vi "User Bridge Control.vi"   [LabVIEW 2011]
uses:
  <vilib>/Rock Robotics/WPI/Solenoid/WPI_SolenoidValue.ctl
  <vilib>/Rock Robotics/WPI/Solenoid/WPI_SolenoidGetEnum.vi
  <vilib>/Rock Robotics/WPI/Solenoid/WPI_SolenoidSetEnum.vi
types:
  T1 = typedef "WPI_JoystickDevRef.ctl" = cluster{"Device":T2}
  T2 = typedef "WPI_JoystickDeviceEnum.ctl" = enum16{"USB 1", "USB 2", "USB 3", "USB 4", "Kinect 1", "Kinect 2"}
  T3 = typedef "WPI_SolenoidDevRef.ctl" = cluster{"DevStatus":errorcluster, "Solenoid Module":T4, "Forward Solenoid Channel":T5, "Reverse Solenoid Channel":T5}
  T4 = typedef "FPGA_TypedefSolenoidModule.ctl" = enum16{"Solenoid Module 1", "Solenoid Module 2"}
  T5 = typedef "WPI_SolenoidChannel.ctl" = enum8{"Solenoid 1", "Solenoid 2", "Solenoid 3", "Solenoid 4", "Solenoid 5", "Solenoid 6", "Solenoid 7", "Solenoid 8", "Invalid"}
  T6 = typedef "WPI_JoystickButtonState.ctl" = cluster{"Button 1":bool, "Button 2":bool, "Button 3":bool, "Button 4":bool, "Button 5":bool, "Button 6":bool, "Button 7":bool, "Button 8":bool, "Button 9":bool, "Button 10":bool, "Button 11":bool, "Button 12":bool}
  T7 = typedef "WPI_SolenoidValue.ctl" = enum16{"Off", "On", "Forward", "Reverse"}
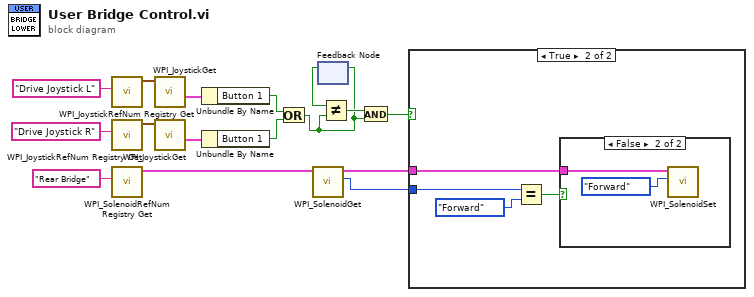
[diagram p0: block diagram]
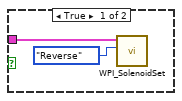
[diagram p3: hidden frame]
diagram:
  n1 = call <vilib>:"WPI_JoystickRefNum Registry Get.vi"("refnum name"="Drive Joystick L") -> ("JoystickDevRef"=w12:T1)  [unwired: 9 in, 1 out]
  n2 = call <vilib>:"WPI_JoystickRefNum Registry Get.vi"("refnum name"="Drive Joystick R") -> ("JoystickDevRef"=w15:T1)  [unwired: 9 in, 1 out]
  n3 = call <vilib>:"WPI_SolenoidRefNum Registry Get.vi"("refnum name"="Rear Bridge") -> ("SolenoidDevRef"=w3:T3)  [unwired: 9 in, 1 out]
  n4 = call <vilib>:"WPI_JoystickGet.vi"("JoystickDevRef"=w12) -> ("Buttons"=w10:T6)  [unwired: 4 in, 2 out]
  n5 = call <vilib>:"WPI_JoystickGet.vi"("JoystickDevRef"=w15) -> ("Buttons"=w14:T6)  [unwired: 4 in, 2 out]
  n6 = Unbundle By Name(w10) -> ("Button 1"=w9:bool)
  n7 = Unbundle By Name(w14) -> ("Button 1"=w8:bool)
  n8 = Or(x=w9, y=w8) -> (x .or. y?=w5:bool)
  n9 = call-poly <vilib>:"WPI_SolenoidGet.vi"("SolenoidDevRef"=w3) -> ("Value"=w1:T7, "SolenoidDevRef"=w2:T3)  [unwired: 8 in, 1 out]
  n10 = feedback-in #1(w5) -> ()
  n11 = feedback #1() -> (w7:bool)  [unwired: 1 in]
  n12 = Not Equal?(x=w7, y=w5) -> (x != y?=w6:bool)
  n13 = And(x=w6, y=w5) -> (x .and. y?=w4:bool)
  n14 = case shown="True" w4 {
    tunnel: w2 -> [_ w20]
    tunnel: w1 -> [_ w19]
    frame False {
    }
    frame True {
      n15 = Equal?(x=w19, y=WPI_SolenoidValue."Forward") -> (x = y?=w17:bool)
      n16 = case shown="False" w17 {
        tunnel: w20 -> [w22 w24]
        frame True {
          n17 = call-poly <vilib>:"WPI_SolenoidSet.vi"("Value"=WPI_SolenoidValue."Reverse", "SolenoidDevRef"=w22) -> ()  [unwired: 8 in, 2 out]
        }
        frame False {
          n18 = call-poly <vilib>:"WPI_SolenoidSet.vi"("Value"=WPI_SolenoidValue."Forward", "SolenoidDevRef"=w24) -> ()  [unwired: 8 in, 2 out]
        }
      }
    }
  }
